vi "AIM664 BITE Transfer.vi"() -> ()   [LabVIEW 2020]
uses:
  AIM664LV.lvlib
panel:
  out "error out":errorcluster
  in  "ClientInfo":T1={"SrvName"="local", "ClHostName"="test", "ClUser"="mr", "ClApplication"="test", "ClApplicationVersion"="1", "ResourceID"=1, "Privileges"=4294967295} {"Privileges" items=["PRIVILEGES_ADMIN"=4294967295]}
  out "NuOfServers":u32=1
  # "ARINC 664 BITE Transfer Test"
  # "Overview: Performs some transfer tests using available port resources of one FDX board. This function will determine the number of ports on the board. If only two ports, it will test them against each other. If four ports are used, Port 1 and Port 2 will be tested against each other and Port 3 and Port 4 will be tested against each other. \nPort 1 and Port 2 must be connected with a Loop-Back cable (crossover), if available Port 3 and Port 4 must be connected with a Loop-Back cable (crossover).\nThe resources of the board under test shall be not logged in.\n\nRequirement: One AIM ARINC-664 board with installed AIM ARINC 664 BSP.\nRestrictions: None.\nInstruction:\n1. Select the Board ID (0 if you have only one board in your system).\n2. Run the VI.\n3. If no error is presented, the test was performed correctly."
  # "FdxInitCvi"
  # "FdxLogoutCvi"
  # "FdxLoginCvi"
  # "FdxBiteTransferCvi"
  # "Input"
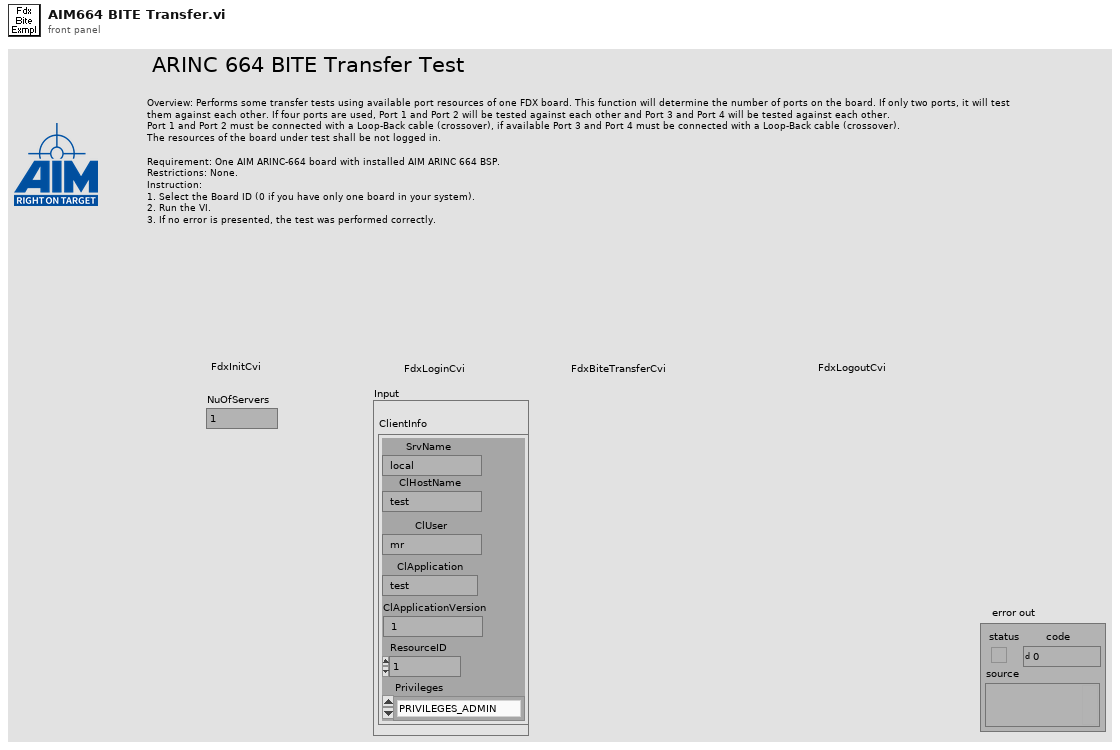
[diagram p1: front panel]
types:
  T1 = cluster{"SrvName":string, "ClHostName":string, "ClUser":string, "ClApplication":string, "ClApplicationVersion":string, "ResourceID":u32, "Privileges":u32}
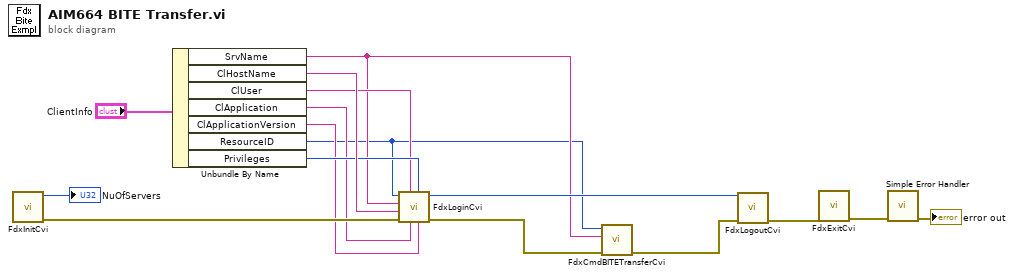
[diagram p0: block diagram]
diagram:
  n1 = call "FdxInitCvi.vi"() -> ("error out"=w15:errorcluster, "Number of Servers"=→"NuOfServers":u32)  [unwired: 10 in]
  n2 = Unbundle By Name("ClientInfo") -> ("SrvName"=w4:string, "ClHostName"=w9:string, "ClUser"=w7:string, "ClApplication"=w6:string, "ClApplicationVersion"=w5:string, "ResourceID"=w3:u32, "Privileges"=w8:u32)
  n3 = call "FdxLoginCvi.vi"("ClApplicationVersion"=w5, "Privileges"=w8, "ClApplication"=w6, "ClUser"=w7, "error in"=w15, "ClHostName"=w9, "SrvName"=w4, "ResourceID"=w3) -> ("error out"=w16:errorcluster, "InstrumentHandle"=w12:u32)  [unwired: 2 in]
  n4 = call "FdxCmdBITETransferCvi.vi"("error in"=w16, "SrvName"=w4, "Board_ResourceID"=w3) -> ("error out"=w14:errorcluster)  [unwired: 7 in, 1 out]
  n5 = call "FdxLogoutCvi.vi"("error in"=w14, "InstrumentHandle"=w12) -> ("error out"=w13:errorcluster)  [unwired: 9 in]
  n6 = call "FdxExitCvi.vi"("error in"=w13) -> ("error out"=w2:errorcluster)  [unwired: 10 in]
  n7 = call <vilib>:"Simple Error Handler.vi"("error in (no error)"=w2) -> ("error out"=→"error out":errorcluster)  [unwired: 4 in, 4 out]
